vi "RWwrapper_setgs.vi"(0 "Strings in":string[](array[string])=["C:\\CuspControl\\GPIB and Network\\Cusp\\u5wavefactoryname.txt", "6723"], 1 "Dubs in":dbl[](array[numeric])=[100000.0, 5.0, 1.0, 0.01, 90.0]) -> ()   [LabVIEW 2018]
panel:
  out "RW on":bool
  in  "RW setgs":T1={"Start Frequency"=100000.0, "Stop Frequency"=100000.0, "Sweep Time"=5.0, "Amplitude"=1.0, "Phase (ch.1)"=0.01, "Phase (Ch.2)"=90.0} {"Sweep Time" format="%.4f"; "Phase (Ch.2)" min=-1800.0 max=1800.0 step=0.1 format="%.3f"; "Phase (ch.1)" min=-1800.0 max=1800.0 step=0.1 format="%.3f"; "Stop Frequency" format="%^.5e"; "Start Frequency" format="%^.5e"; "Amplitude" min=0.0 max=4.0 format="%.3f"}
  out "VISAsession":string="wavefactoryU5"
  in  "Synth names file":path=path "C:/CuspControl/GPIB and Network/Cusp/u5wavefactoryname.txt"
  in  "subvi":bool=TRUE
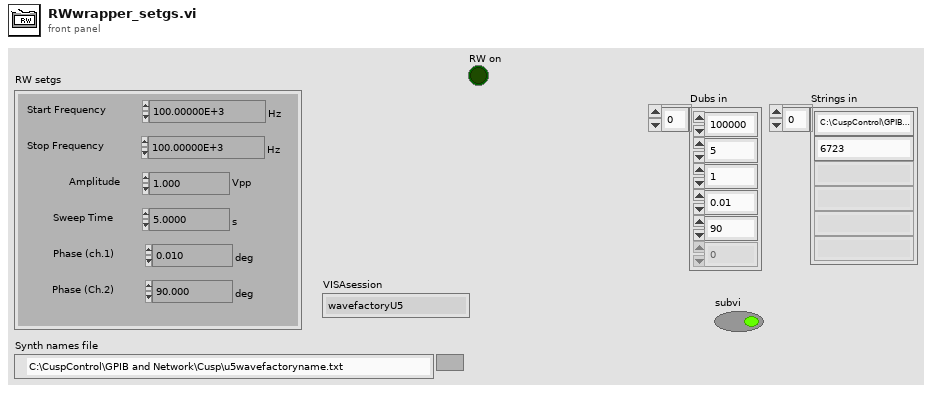
[diagram p1: front panel]
types:
  T1 = cluster{"Start Frequency":dbl, "Stop Frequency":dbl, "Sweep Time":dbl, "Amplitude":dbl, "Phase (ch.1)":dbl, "Phase (Ch.2)":dbl}
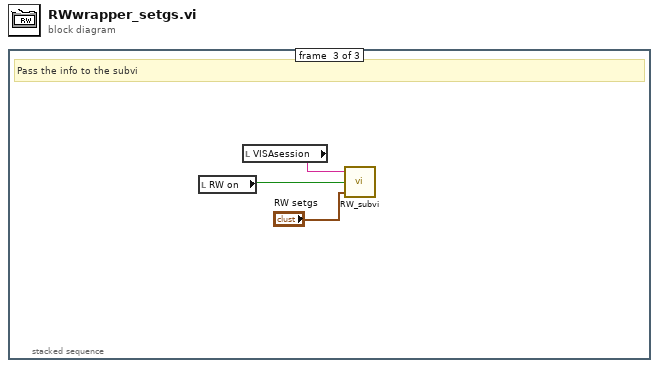
[diagram p0: block diagram]
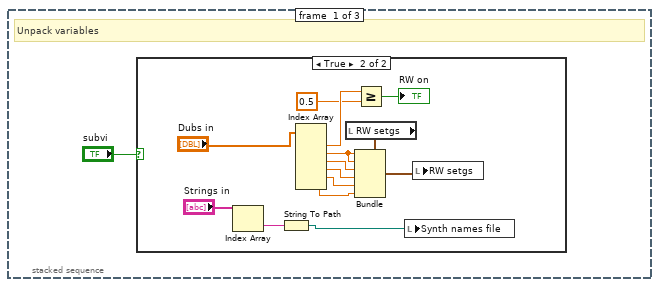
[diagram p2: hidden frame]
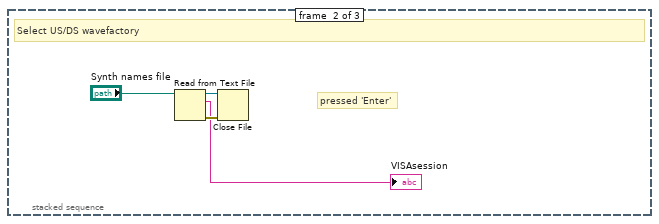
[diagram p4: hidden frame]
diagram:
  n1 = stacked-sequence {
    frame #0 {
      # "Unpack variables"
      n2 = case shown="True" "subvi" {
        frame False {
        }
        frame True {
          n3 = Index Array(array="Strings in") -> (element=w14:string)  [unwired: 1 in]
          n4 = String To Path(string=w14) -> (path=w13:path)
          n5 = Index Array(array="Dubs in") -> (element #1=w4:dbl, element #2=w12:dbl, element #3=w8:dbl, element #4=w7:dbl, element #5=w6:dbl, element #6=w5:dbl)  [unwired: 6 in]
          n6 = local read "RW setgs"() -> (w10:T1)
          n7 = Bundle(cluster=w10, "Start Frequency"=w12, "Stop Frequency"=w12, "Sweep Time"=w8, "Amplitude"=w7, "Phase (ch.1)"=w6, "Phase (Ch.2)"=w5) -> (w9:T1)
          n8 = Greater Or Equal?(x=w4, y=0.5) -> (x >= y?=→"RW on":bool)
          n9 = local write "Synth names file"(w13) -> ()
          n10 = local write "RW setgs"(w9) -> ()
        }
      }
    }
    frame #1 {
      # "pressed 'Enter'"
      # "Select US/DS wavefactory"
      n11 = Read from Text File(file (use dialog)="Synth names file") -> (refnum out=w17:refnum<file>, text=→"VISAsession":string, error out=w18:errorcluster)  [unwired: 3 in, 1 out]
      n12 = Close File(refnum=w17, error in=w18) -> ()  [unwired: 2 out]
    }
    frame #2 {
      # "Pass the info to the subvi"
      n13 = local read "RW on"() -> (w20:bool)
      n14 = local read "VISAsession"() -> (w22:string)
      n15 = call "RW_subvi.vi"("Rotating Wall Parameters"="RW setgs", "On/Off"=w20, "VISAsession"=w22) -> ()
    }
  }
